vi "RN_20.vi"(8 "error in (no error)":errorcluster, 11 "NN in":T1={"Name"="Name", "No of Layers"=0, "mBatch"=0, "Layers"=[], "Dimty"=enum."In1D_Out1D", "Dims_In"={"C"=0, "H"=0, "W"=0}, "Dims_Out"={"C"=0, "H"=0, "W"=0}, "Working_Dir"=path "", "Train?"=FALSE, "Train_Params"={"Optimizer"=enum."SGD", "Beta_1"=0.0, "Beta_2"=0.0, "Weight Decay(L1)"=0.0, "Weight Decay(L2)"=0.0, "Data_Sampling"=enum."Random"}, "LR_Update_Policy"={"Policy_Type"=enum."Manual", "LR0"=0.0, "k"=0.0, "WarmUp_Policy"=enum."Step", "WarmUp_Iter"=100, "WarmUp_Ratio"=10.0}, "Session Data"={"Epochs"=0.0, "Tot_Iter"=0, "LR"=0.0, "LR_iter"=0}, "Ground_truth"={"Y"=variant(refnum<data-value> refnum)}, "NNg_hdls"={"cudnn"=0, "cublas"=0, "stream"=0, "curand"=0}, "NN_Device"=enum."CPU", "GPU Id"=0, "Labels"=[], "Receptive Field"=[], "Loss_Type"=enum."MSE", "Loss_Cfg_Prms"=variant, "NNG_WS"={"NNG_WS_Mem"=refnum, "Max_WS_Size"=0}} {"LR_Update_Policy"."WarmUp_Ratio" min=1; "LR_Update_Policy"."WarmUp_Iter" min=1; "LR_Update_Policy"."LR0" format="%.7f"}) -> (0 "error out":errorcluster, 3 "NN out":T1={"Name"="Name", "No of Layers"=0, "mBatch"=0, "Layers"=[], "Dimty"=enum."In1D_Out1D", "Dims_In"={"C"=0, "H"=0, "W"=0}, "Dims_Out"={"C"=0, "H"=0, "W"=0}, "Working_Dir"=path "", "Train?"=FALSE, "Train_Params"={"Optimizer"=enum."SGD", "Beta_1"=0.0, "Beta_2"=0.0, "Weight Decay(L1)"=0.0, "Weight Decay(L2)"=0.0, "Data_Sampling"=enum."Random"}, "LR_Update_Policy"={"Policy_Type"=enum."Manual", "LR0"=0.0, "k"=0.0, "WarmUp_Policy"=enum."Step", "WarmUp_Iter"=100, "WarmUp_Ratio"=10.0}, "Session Data"={"Epochs"=0.0, "Tot_Iter"=0, "LR"=0.0, "LR_iter"=0}, "Ground_truth"={"Y"=variant(refnum<data-value> refnum)}, "NNg_hdls"={"cudnn"=0, "cublas"=0, "stream"=0, "curand"=0}, "NN_Device"=enum."CPU", "GPU Id"=0, "Labels"=[], "Receptive Field"=[], "Loss_Type"=enum."MSE", "Loss_Cfg_Prms"=variant, "NNG_WS"={"NNG_WS_Mem"=refnum, "Max_WS_Size"=0}} {"LR_Update_Policy"."WarmUp_Ratio" min=1; "LR_Update_Policy"."WarmUp_Iter" min=1; "LR_Update_Policy"."LR0" format="%.7f"})   [LabVIEW 2020]
uses:
  <vilib>/Ngene/Deep Learning Toolkit/Toolkit/NN_Network/Controls/NN.ctl
  <vilib>/Ngene/Deep Learning Toolkit/Toolkit/NN_Layers/Controls/NN_Layer_ref.ctl
  <vilib>/Ngene/Deep Learning Toolkit/Toolkit/NN_Layers/Controls/NN_Layer.ctl
  <vilib>/Ngene/Deep Learning Toolkit/Toolkit/NN_Layers/Controls/NN_Layer_Type.ctl
  <vilib>/Ngene/Deep Learning Toolkit/Toolkit/NN_Data/API/NN_Dims(C,H,W).ctl
  <vilib>/Ngene/Deep Learning Toolkit/Toolkit/NN_Layers/Controls/NN_Layer_Metrics.ctl
  <vilib>/Ngene/Deep Learning Toolkit/Toolkit/NN_Network/Controls/NN_Device.ctl
  <vilib>/Ngene/Deep Learning Toolkit/Toolkit/NNg/cuda/Controls/nng_cuda_handles.ctl
  <vilib>/Ngene/Deep Learning Toolkit/Toolkit/NN_Layers/Controls/NN_Layer_Dimty.ctl
  <vilib>/Ngene/Deep Learning Toolkit/Toolkit/NN_Layers/Controls/NN_Layer_RF_State.ctl
  <vilib>/Ngene/Deep Learning Toolkit/Toolkit/NN_Data/API/NN_Dims(V,H).ctl
  <vilib>/Ngene/Deep Learning Toolkit/Toolkit/NN_Network/Controls/NN_In_Out_Dim-ty.ctl
  <vilib>/Ngene/Deep Learning Toolkit/Toolkit/NN_Train/Controls/NN_Train_Params.ctl
  <vilib>/Ngene/Deep Learning Toolkit/Toolkit/NN_Train/Controls/NN_Train_Optimizer.ctl
  <vilib>/Ngene/Deep Learning Toolkit/Toolkit/NN_Train/Controls/NN_Train_Data_Sampling.ctl
  <vilib>/Ngene/Deep Learning Toolkit/Toolkit/NN_Train/Controls/NN_LR_Policy_Cfg.ctl
  <vilib>/Ngene/Deep Learning Toolkit/Toolkit/NN_Train/Controls/NN_LR_Policy_Type.ctl
  <vilib>/Ngene/Deep Learning Toolkit/Toolkit/NN_Train/Controls/NN_Train_Session_Data.ctl
  <vilib>/Ngene/Deep Learning Toolkit/Toolkit/NN_Data/Controls/NN_Ground_truth.ctl
  <vilib>/Ngene/Deep Learning Toolkit/Toolkit/NN_Train/Controls/NN_Loss_Type.ctl
  <vilib>/Ngene/Deep Learning Toolkit/Toolkit/NNg/Network/WS/Controls/NNG_WS.ctl
  <vilib>/Ngene/Deep Learning Toolkit/Toolkit/NNg/Network/WS/Controls/NNg_WS_Mem_DVR.ctl
  <vilib>/Ngene/Deep Learning Toolkit/Toolkit/NNg/cuda/Controls/cuda_Mem_desc.ctl
  <vilib>/Ngene/Deep Learning Toolkit/Toolkit/NN_Layers/Layers/Conv2D/Controls/NN_Layer_Config(Conv2D).ctl
  <vilib>/Ngene/Deep Learning Toolkit/Toolkit/NN_Layers/Layers/Conv2D/Controls/NN_Layer_Params(Conv2D).ctl
  <vilib>/Ngene/Deep Learning Toolkit/Toolkit/NN_Layers/Layers/Conv2D/Controls/NN_Conv2D_Padding_Type.ctl
  <vilib>/Ngene/Deep Learning Toolkit/Toolkit/NN_Layers/Layers/BatchNorm/Controls/NN_BN_Params.ctl
  <vilib>/Ngene/Deep Learning Toolkit/Toolkit/NN_Activations/Controls/NN_Activation_Type.ctl
  <vilib>/Ngene/Deep Learning Toolkit/Toolkit/NN_Layers/Controls/NN_Layer_Init_Params.ctl
  <vilib>/Ngene/Deep Learning Toolkit/Toolkit/NN_Layers/Controls/NN_Layer_Weight_Init_Type.ctl
  <vilib>/Ngene/Deep Learning Toolkit/Toolkit/NN_Layers/Layers/ShortCut/Controls/NN_Layer_Config(ShortCut).ctl
  <vilib>/Ngene/Deep Learning Toolkit/Toolkit/NN_Layers/Layers/Pool/Controls/NN_Layer_Config(Pool).ctl
  <vilib>/Ngene/Deep Learning Toolkit/Toolkit/NN_Layers/Layers/Conv2D/NN_Layer_Create(Conv2D).vi
  <vilib>/Ngene/Deep Learning Toolkit/Toolkit/NN_Layers/Layers/ShortCut/NN_Layer_Create(ShortCut).vi
  <vilib>/Ngene/Deep Learning Toolkit/Toolkit/NN_Layers/Layers/Pool/NN_Layer_Create(avgPool).vi
  <vilib>/Ngene/Deep Learning Toolkit/Toolkit/Deep_Learning_Toolkit_by_Ngene.lvlib
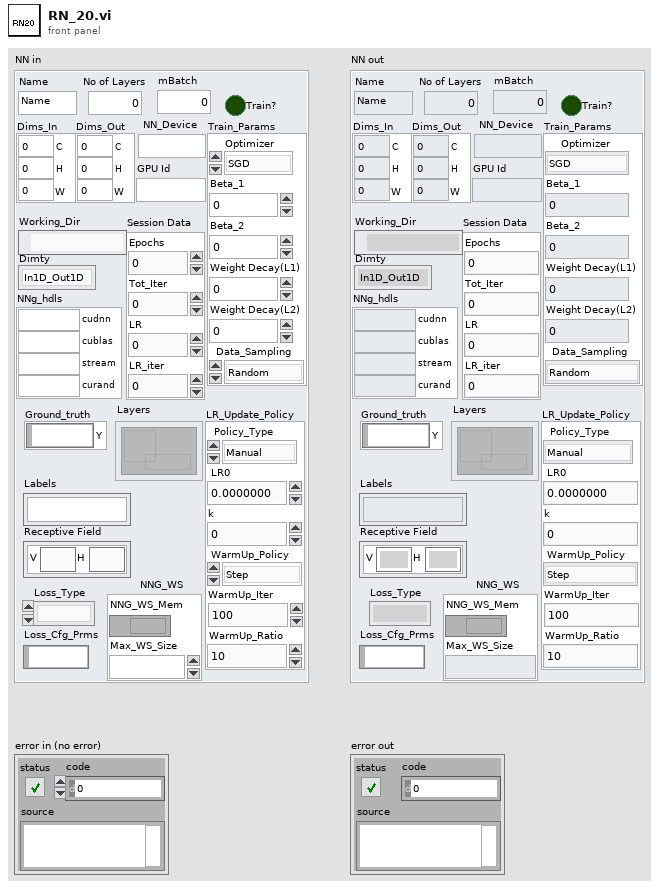
[diagram p1: front panel]
types:
  T1 = typedef "Deep_Learning_Toolkit_by_Ngene.lvlib/NN.ctl" = cluster{"Name":string, "No of Layers":i32, "mBatch":i32, "Layers":T2[], "Dimty":T3, "Dims_In":T4, "Dims_Out":T4, "Working_Dir":path, "Train?":bool, "Train_Params":T5, "LR_Update_Policy":T8, "Session Data":T10, "Ground_truth":T11, "NNg_hdls":T12, "NN_Device":T13, "GPU Id":i32, "Labels":string[], "Receptive Field":T14[], "Loss_Type":T15, "Loss_Cfg_Prms":variant, "NNG_WS":T16}
  T2 = typedef "Deep_Learning_Toolkit_by_Ngene.lvlib/NN_Layer_ref.ctl" = refnum<data-value>
  T3 = typedef "Deep_Learning_Toolkit_by_Ngene.lvlib/NN_In_Out_Dim-ty.ctl" = enum8{"In1D_Out1D", "In3D_Out1D", "In3D_Out3D", "In3D_OutBBox"}
  T4 = typedef "Deep_Learning_Toolkit_by_Ngene.lvlib/NN_Dims(C,H,W).ctl" = cluster{"C":i32, "H":i32, "W":i32}
  T5 = typedef "Deep_Learning_Toolkit_by_Ngene.lvlib/NN_Train_Params.ctl" = cluster{"Optimizer":T6, "Beta_1":sgl, "Beta_2":sgl, "Weight Decay(L1)":sgl, "Weight Decay(L2)":sgl, "Data_Sampling":T7}
  T6 = typedef "Deep_Learning_Toolkit_by_Ngene.lvlib/NN_Train_Optimizer.ctl" = enum16{"SGD", "Adam", "Adagrad", "Adadelta", "RMSProp", "Nesterov"}
  T7 = typedef "Deep_Learning_Toolkit_by_Ngene.lvlib/NN_Train_Data_Sampling.ctl" = enum16{"Random", "Sequential"}
  T8 = typedef "Deep_Learning_Toolkit_by_Ngene.lvlib/NN_LR_Policy_Cfg.ctl" = cluster{"Policy_Type":T9, "LR0":dbl, "k":sgl, "WarmUp_Policy":enum16{"Step", "Ramp"}, "WarmUp_Iter":i32, "WarmUp_Ratio":sgl}
  T9 = typedef "Deep_Learning_Toolkit_by_Ngene.lvlib/NN_LR_Policy_Type.ctl" = enum16{"Manual", "Step", "Exp", "1/t"}
  T10 = typedef "Deep_Learning_Toolkit_by_Ngene.lvlib/NN_Train_Session_Data.ctl" = cluster{"Epochs":sgl, "Tot_Iter":i32, "LR":sgl, "LR_iter":i32}
  T11 = typedef "Deep_Learning_Toolkit_by_Ngene.lvlib/NN_Ground_truth.ctl" = cluster{"Y":variant}
  T12 = typedef "Deep_Learning_Toolkit_by_Ngene.lvlib/nng_cuda_handles.ctl" = cluster{"cudnn":u64, "cublas":u64, "stream":u64, "curand":u64}
  T13 = typedef "Deep_Learning_Toolkit_by_Ngene.lvlib/NN_Device.ctl" = enum16{"CPU", "GPU"}
  T14 = typedef "Deep_Learning_Toolkit_by_Ngene.lvlib/NN_Dims(V,H).ctl" = cluster{"V":i32, "H":i32}
  T15 = typedef "Deep_Learning_Toolkit_by_Ngene.lvlib/NN_Loss_Type.ctl" = enum16{"None", "MSE", "CrossEntropy", "YOLO_v2", "YOLO_v4"}
  T16 = typedef "Deep_Learning_Toolkit_by_Ngene.lvlib/NNG_WS.ctl" = cluster{"NNG_WS_Mem":T17, "Max_WS_Size":i64}
  T17 = typedef "Deep_Learning_Toolkit_by_Ngene.lvlib/NNg_WS_Mem_DVR.ctl" = refnum<data-value>
  T18 = typedef "Deep_Learning_Toolkit_by_Ngene.lvlib/NN_Layer_Config(Pool).ctl" = cluster{"Name":string, "Size":T14, "Stride":T14, "Pad_Type":T19, "Pad_Size":T14}
  T19 = typedef "Deep_Learning_Toolkit_by_Ngene.lvlib/NN_Conv2D_Padding_Type.ctl" = enum16{"Pad_Size", "Valid", "Same"}
  T20 = typedef "Deep_Learning_Toolkit_by_Ngene.lvlib/NN_Layer_Config(ShortCut).ctl" = cluster{"Name":string, "Activation":T21}
  T21 = typedef "Deep_Learning_Toolkit_by_Ngene.lvlib/NN_Activation_Type.ctl" = enum16{"Sigmoid", "ReLU", "LReLU", "ReLU6", "tanh", "Swish", "Mish", "None"}
  T22 = typedef "Deep_Learning_Toolkit_by_Ngene.lvlib/NN_Layer_Config(Conv2D).ctl" = cluster{"Name":string, "Conv_Params":T23, "BN?":bool, "BN_Params":T24, "Activation":T21, "Has Bias?":bool, "Init_Params":T25, "Custom_Params":string}
  T23 = typedef "Deep_Learning_Toolkit_by_Ngene.lvlib/NN_Layer_Params(Conv2D).ctl" = cluster{"Filters":i32, "Kernel_Size":i32, "Stride":i32, "Pad_Type":T19, "Pad_Size":i32}
  T24 = typedef "Deep_Learning_Toolkit_by_Ngene.lvlib/NN_BN_Params.ctl" = cluster{"epsilon":sgl, "momentum":sgl}
  T25 = typedef "Deep_Learning_Toolkit_by_Ngene.lvlib/NN_Layer_Init_Params.ctl" = cluster{"Init_Type":T26, "Value":sgl}
  T26 = typedef "Deep_Learning_Toolkit_by_Ngene.lvlib/NN_Layer_Weight_Init_Type.ctl" = enum16{"Const", "Uniform", "Gaussian", "Xavier"}
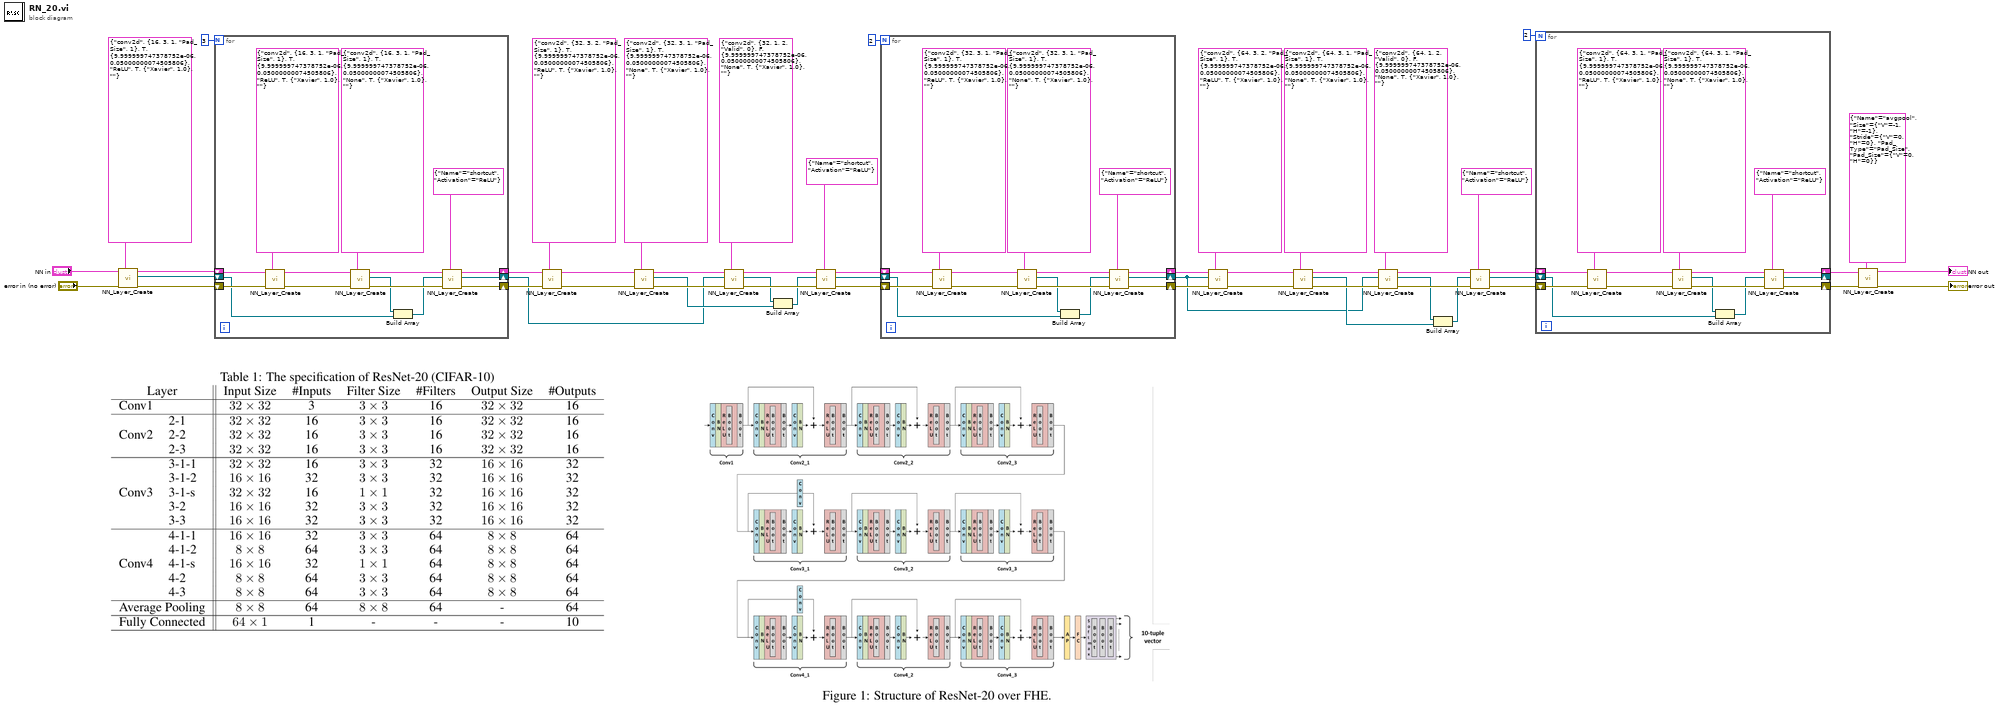
[diagram p0: block diagram]
diagram:
  n1 = call-poly <vilib>:"NN_Layer_Create.vi"("Conv2D_Cfg"=T22 {"Name"="conv2d", "Conv_Params"={"Filters"=16, "Kernel_Size"=3, "Stride"=1, "Pad_Type"=enum."Pad_Size", "Pad_Size"=1}, "BN?"=TRUE, "BN_Params"={"epsilon"=1e-05, "momentum"=0.05}, "Activation"=enum."ReLU", "Has Bias?"=TRUE, "Init_Params"={"Init_Type"=enum."Xavier", "Value"=1.0}, "Custom_Params"=""} ("Conv2D_Config"), "error in (no error)"="error in (no error)", "NN in"="NN in") -> ("error out"=w50:errorcluster, "Layer_Out"=w47:T2, "NN out"=w51:T1)  [unwired: 6 in]
  n2 = for {
    N: 3 -> [_]
    shift-right: [w58] -> w32
    shift-left: w51 -> [w64]
    shift-right: [w57] -> w31
    shift-left: w50 -> [w63]
    shift-right: [w53] -> w30
    shift-left: w47 -> [w54]
    n3 = call-poly <vilib>:"NN_Layer_Create.vi"("Conv2D_Cfg"=T22 {"Name"="conv2d", "Conv_Params"={"Filters"=16, "Kernel_Size"=3, "Stride"=1, "Pad_Type"=enum."Pad_Size", "Pad_Size"=1}, "BN?"=TRUE, "BN_Params"={"epsilon"=1e-05, "momentum"=0.05}, "Activation"=enum."ReLU", "Has Bias?"=TRUE, "Init_Params"={"Init_Type"=enum."Xavier", "Value"=1.0}, "Custom_Params"=""} ("Conv2D_Config"), "error in (no error)"=w63, "NN in"=w64) -> ("error out"=w61:errorcluster, "NN out"=w62:T1)  [unwired: 6 in, 1 out]
    n4 = call-poly <vilib>:"NN_Layer_Create.vi"("Conv2D_Cfg"=T22 {"Name"="conv2d", "Conv_Params"={"Filters"=16, "Kernel_Size"=3, "Stride"=1, "Pad_Type"=enum."Pad_Size", "Pad_Size"=1}, "BN?"=TRUE, "BN_Params"={"epsilon"=1e-05, "momentum"=0.05}, "Activation"=enum."None", "Has Bias?"=TRUE, "Init_Params"={"Init_Type"=enum."Xavier", "Value"=1.0}, "Custom_Params"=""} ("Conv2D_Config"), "error in (no error)"=w61, "NN in"=w62) -> ("error out"=w59:errorcluster, "Layer_Out"=w56:T2, "NN out"=w60:T1)  [unwired: 6 in]
    n5 = Build Array(w56, w54) -> (w55:T2[])
    n6 = call-poly <vilib>:"NN_Layer_Create.vi"("ShortCut_Cfg"=T20 {"Name"="shortcut", "Activation"=enum."ReLU"} ("ShortCut Config Params"), "error in (no error)"=w59, "Input_Layer_Refs"=w55, "NN in"=w60) -> ("error out"=w57:errorcluster, "Layer_Out"=w53:T2, "NN out"=w58:T1)  [unwired: 5 in]
  }
  n7 = call-poly <vilib>:"NN_Layer_Create.vi"("Conv2D_Cfg"=T22 {"Name"="conv2d", "Conv_Params"={"Filters"=32, "Kernel_Size"=3, "Stride"=2, "Pad_Type"=enum."Pad_Size", "Pad_Size"=1}, "BN?"=TRUE, "BN_Params"={"epsilon"=1e-05, "momentum"=0.05}, "Activation"=enum."ReLU", "Has Bias?"=TRUE, "Init_Params"={"Init_Type"=enum."Xavier", "Value"=1.0}, "Custom_Params"=""} ("Conv2D_Config"), "error in (no error)"=w31, "NN in"=w32) -> ("error out"=w40:errorcluster, "NN out"=w41:T1)  [unwired: 6 in, 1 out]
  n8 = call-poly <vilib>:"NN_Layer_Create.vi"("Conv2D_Cfg"=T22 {"Name"="conv2d", "Conv_Params"={"Filters"=32, "Kernel_Size"=3, "Stride"=1, "Pad_Type"=enum."Pad_Size", "Pad_Size"=1}, "BN?"=TRUE, "BN_Params"={"epsilon"=1e-05, "momentum"=0.05}, "Activation"=enum."None", "Has Bias?"=TRUE, "Init_Params"={"Init_Type"=enum."Xavier", "Value"=1.0}, "Custom_Params"=""} ("Conv2D_Config"), "error in (no error)"=w40, "NN in"=w41) -> ("error out"=w38:errorcluster, "Layer_Out"=w34:T2, "NN out"=w39:T1)  [unwired: 6 in]
  n9 = call-poly <vilib>:"NN_Layer_Create.vi"("Conv2D_Cfg"=T22 {"Name"="conv2d", "Conv_Params"={"Filters"=32, "Kernel_Size"=1, "Stride"=2, "Pad_Type"=enum."Valid", "Pad_Size"=0}, "BN?"=FALSE, "BN_Params"={"epsilon"=1e-05, "momentum"=0.05}, "Activation"=enum."None", "Has Bias?"=TRUE, "Init_Params"={"Init_Type"=enum."Xavier", "Value"=1.0}, "Custom_Params"=""} ("Conv2D_Config"), "error in (no error)"=w38, "Input_Layer"=w30, "NN in"=w39) -> ("error out"=w36:errorcluster, "Layer_Out"=w35:T2, "NN out"=w37:T1)  [unwired: 5 in]
  n10 = Build Array(w35, w34) -> (w33:T2[])
  n11 = call-poly <vilib>:"NN_Layer_Create.vi"("ShortCut_Cfg"=T20 {"Name"="shortcut", "Activation"=enum."ReLU"} ("ShortCut Config Params"), "error in (no error)"=w36, "Input_Layer_Refs"=w33, "NN in"=w37) -> ("error out"=w28:errorcluster, "Layer_Out"=w27:T2, "NN out"=w29:T1)  [unwired: 5 in]
  n12 = for {
    N: 2 -> [_]
    shift-right: [w73] -> w8
    shift-left: w29 -> [w79]
    shift-right: [w72] -> w7
    shift-left: w28 -> [w78]
    shift-right: [w68] -> w6
    shift-left: w27 -> [w69]
    n13 = call-poly <vilib>:"NN_Layer_Create.vi"("Conv2D_Cfg"=T22 {"Name"="conv2d", "Conv_Params"={"Filters"=32, "Kernel_Size"=3, "Stride"=1, "Pad_Type"=enum."Pad_Size", "Pad_Size"=1}, "BN?"=TRUE, "BN_Params"={"epsilon"=1e-05, "momentum"=0.05}, "Activation"=enum."ReLU", "Has Bias?"=TRUE, "Init_Params"={"Init_Type"=enum."Xavier", "Value"=1.0}, "Custom_Params"=""} ("Conv2D_Config"), "error in (no error)"=w78, "NN in"=w79) -> ("error out"=w76:errorcluster, "NN out"=w77:T1)  [unwired: 6 in, 1 out]
    n14 = call-poly <vilib>:"NN_Layer_Create.vi"("Conv2D_Cfg"=T22 {"Name"="conv2d", "Conv_Params"={"Filters"=32, "Kernel_Size"=3, "Stride"=1, "Pad_Type"=enum."Pad_Size", "Pad_Size"=1}, "BN?"=TRUE, "BN_Params"={"epsilon"=1e-05, "momentum"=0.05}, "Activation"=enum."None", "Has Bias?"=TRUE, "Init_Params"={"Init_Type"=enum."Xavier", "Value"=1.0}, "Custom_Params"=""} ("Conv2D_Config"), "error in (no error)"=w76, "NN in"=w77) -> ("error out"=w74:errorcluster, "Layer_Out"=w71:T2, "NN out"=w75:T1)  [unwired: 6 in]
    n15 = Build Array(w71, w69) -> (w70:T2[])
    n16 = call-poly <vilib>:"NN_Layer_Create.vi"("ShortCut_Cfg"=T20 {"Name"="shortcut", "Activation"=enum."ReLU"} ("ShortCut Config Params"), "error in (no error)"=w74, "Input_Layer_Refs"=w70, "NN in"=w75) -> ("error out"=w72:errorcluster, "Layer_Out"=w68:T2, "NN out"=w73:T1)  [unwired: 5 in]
  }
  n17 = call-poly <vilib>:"NN_Layer_Create.vi"("Conv2D_Cfg"=T22 {"Name"="conv2d", "Conv_Params"={"Filters"=64, "Kernel_Size"=3, "Stride"=2, "Pad_Type"=enum."Pad_Size", "Pad_Size"=1}, "BN?"=TRUE, "BN_Params"={"epsilon"=1e-05, "momentum"=0.05}, "Activation"=enum."ReLU", "Has Bias?"=TRUE, "Init_Params"={"Init_Type"=enum."Xavier", "Value"=1.0}, "Custom_Params"=""} ("Conv2D_Config"), "error in (no error)"=w7, "Input_Layer"=w6, "NN in"=w8) -> ("error out"=w20:errorcluster, "NN out"=w21:T1)  [unwired: 5 in, 1 out]
  n18 = call-poly <vilib>:"NN_Layer_Create.vi"("Conv2D_Cfg"=T22 {"Name"="conv2d", "Conv_Params"={"Filters"=64, "Kernel_Size"=3, "Stride"=1, "Pad_Type"=enum."Pad_Size", "Pad_Size"=1}, "BN?"=TRUE, "BN_Params"={"epsilon"=1e-05, "momentum"=0.05}, "Activation"=enum."None", "Has Bias?"=TRUE, "Init_Params"={"Init_Type"=enum."Xavier", "Value"=1.0}, "Custom_Params"=""} ("Conv2D_Config"), "error in (no error)"=w20, "NN in"=w21) -> ("error out"=w18:errorcluster, "Layer_Out"=w14:T2, "NN out"=w19:T1)  [unwired: 6 in]
  n19 = call-poly <vilib>:"NN_Layer_Create.vi"("Conv2D_Cfg"=T22 {"Name"="conv2d", "Conv_Params"={"Filters"=64, "Kernel_Size"=1, "Stride"=2, "Pad_Type"=enum."Valid", "Pad_Size"=0}, "BN?"=FALSE, "BN_Params"={"epsilon"=1e-05, "momentum"=0.05}, "Activation"=enum."None", "Has Bias?"=TRUE, "Init_Params"={"Init_Type"=enum."Xavier", "Value"=1.0}, "Custom_Params"=""} ("Conv2D_Config"), "error in (no error)"=w18, "Input_Layer"=w6, "NN in"=w19) -> ("error out"=w16:errorcluster, "Layer_Out"=w15:T2, "NN out"=w17:T1)  [unwired: 5 in]
  n20 = Build Array(w15, w14) -> (w13:T2[])
  n21 = call-poly <vilib>:"NN_Layer_Create.vi"("ShortCut_Cfg"=T20 {"Name"="shortcut", "Activation"=enum."ReLU"} ("ShortCut Config Params"), "error in (no error)"=w16, "Input_Layer_Refs"=w13, "NN in"=w17) -> ("error out"=w11:errorcluster, "Layer_Out"=w10:T2, "NN out"=w12:T1)  [unwired: 5 in]
  n22 = for {
    N: 2 -> [_]
    shift-right: [w88] -> w4
    shift-left: w12 -> [w94]
    shift-right: [w87] -> w3
    shift-left: w11 -> [w93]
    shift-right: [w83] -> _
    shift-left: w10 -> [w84]
    n23 = call-poly <vilib>:"NN_Layer_Create.vi"("Conv2D_Cfg"=T22 {"Name"="conv2d", "Conv_Params"={"Filters"=64, "Kernel_Size"=3, "Stride"=1, "Pad_Type"=enum."Pad_Size", "Pad_Size"=1}, "BN?"=TRUE, "BN_Params"={"epsilon"=1e-05, "momentum"=0.05}, "Activation"=enum."ReLU", "Has Bias?"=TRUE, "Init_Params"={"Init_Type"=enum."Xavier", "Value"=1.0}, "Custom_Params"=""} ("Conv2D_Config"), "error in (no error)"=w93, "NN in"=w94) -> ("error out"=w91:errorcluster, "NN out"=w92:T1)  [unwired: 6 in, 1 out]
    n24 = call-poly <vilib>:"NN_Layer_Create.vi"("Conv2D_Cfg"=T22 {"Name"="conv2d", "Conv_Params"={"Filters"=64, "Kernel_Size"=3, "Stride"=1, "Pad_Type"=enum."Pad_Size", "Pad_Size"=1}, "BN?"=TRUE, "BN_Params"={"epsilon"=1e-05, "momentum"=0.05}, "Activation"=enum."None", "Has Bias?"=TRUE, "Init_Params"={"Init_Type"=enum."Xavier", "Value"=1.0}, "Custom_Params"=""} ("Conv2D_Config"), "error in (no error)"=w91, "NN in"=w92) -> ("error out"=w89:errorcluster, "Layer_Out"=w86:T2, "NN out"=w90:T1)  [unwired: 6 in]
    n25 = Build Array(w86, w84) -> (w85:T2[])
    n26 = call-poly <vilib>:"NN_Layer_Create.vi"("ShortCut_Cfg"=T20 {"Name"="shortcut", "Activation"=enum."ReLU"} ("ShortCut Config Params"), "error in (no error)"=w89, "Input_Layer_Refs"=w85, "NN in"=w90) -> ("error out"=w87:errorcluster, "Layer_Out"=w83:T2, "NN out"=w88:T1)  [unwired: 5 in]
  }
  n27 = call-poly <vilib>:"NN_Layer_Create.vi"("AvgPool_Cfg"=T18 {"Name"="avgpool", "Size"={"V"=-1, "H"=-1}, "Stride"={"V"=0, "H"=0}, "Pad_Type"=enum."Pad_Size", "Pad_Size"={"V"=0, "H"=0}} ("Pool Config Params"), "error in (no error)"=w3, "NN in"=w4) -> ("error out"=→"error out":errorcluster, "NN out"=→"NN out":T1)  [unwired: 6 in, 1 out]
